vi "Plot Data.vi"(8 "error in (no error)":errorcluster, 11 "DigitiserActor in":refnum<class "DigitiserActor.lvclass">) -> (0 "error out":errorcluster, 3 "DigitiserActor out":refnum<class "DigitiserActor.lvclass">)   [LabVIEW 2019, in "DigitiserActor.lvlib" / "DigitiserActor.lvclass"]
uses:
  DigitiserActor.lvclass
  C:/Program Files (x86)/National Instruments/LabVIEW 2019/vi.lib/ActorFramework/Actor/Actor.lvclass
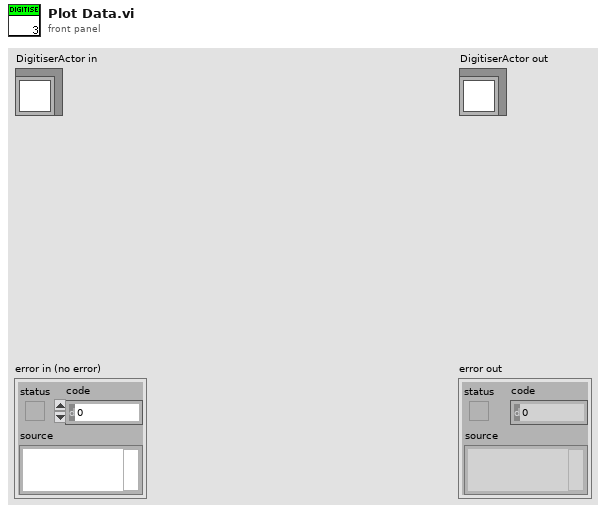
[diagram p1: front panel]
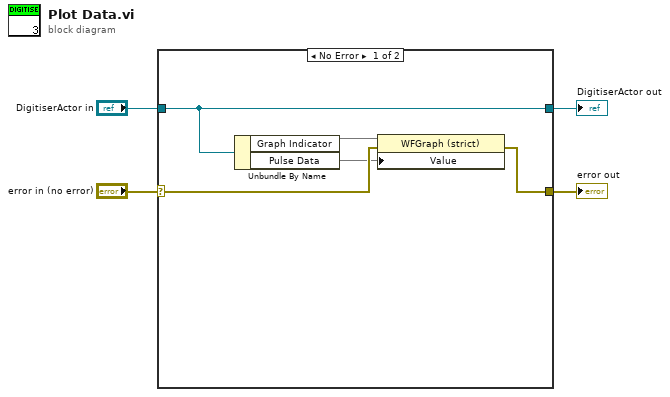
[diagram p0: block diagram]
diagram:
  n1 = case shown="No Error" "error in (no error)" {
    selector: "error in (no error)" -> [w8 w11]
    tunnel: [w7 w11] -> w3
    tunnel: [w9 w10] -> w1
    tunnel: "DigitiserActor in" -> [w9 w10]
    frame No Error {
      n2 = Unbundle By Name(w9) -> ("Graph Indicator"=w6, "Pulse Data"=w5)
      n3 = property class="WFGraph (strict)"(reference=w6, error in=w8, "Value"=w5) -> (error out=w7:errorcluster)  [unwired: 1 out]
    }
    frame Error {
    }
  }
  "error out" <- w3
  "DigitiserActor out" <- w1
